vi "serpenbot_DDPG_learing.vi"() -> ()   [LabVIEW 2020]
uses:
  <vilib>/Analysis/Matrix/Datatypes/RealMatrix.ctl
  <vilib>/Analysis/Matrix/NI_Matrix.lvlib
  <vilib>/Analysis/NI_AALBase.lvlib
  <vilib>/Analysis/baseanly.llb/Real A x B.vi
  <vilib>/Analysis/NI_AALPro.lvlib
  <vilib>/Analysis/_algsub.llb/Real PseudoInverse Matrix.vi
  <vilib>/Analysis/Matrix/Numeric/Subtract/Subtract - RM,RM.vi
  <vilib>/Analysis/Matrix/Numeric/Conversions/Array To Matrix - RA.vi
panel:
  out "error out Y":errorcluster
  out "error out X":errorcluster
  out "laser control value":dbl[](array[numeric])
  out "control_loop_time":u32
  in  "stop":bool
  in  "Logging":bool caption="Enable"
  in  "k":T1
  in  "Diode Current\nSetting":dbl=3.0
  in  "Laser Repetition\nFrequency":i32=50000
  in  "VISA resource name":refnum<visa-resource-name>="COM14"
  in  "baud rate (9600)":u32=9600
  out "error out":errorcluster
  out "Identification system 1":string
  out "Conn. axes system 1":string[](array[string])
  out "Identification system 2":string
  out "Conn. axes system  2":string[](array[string])
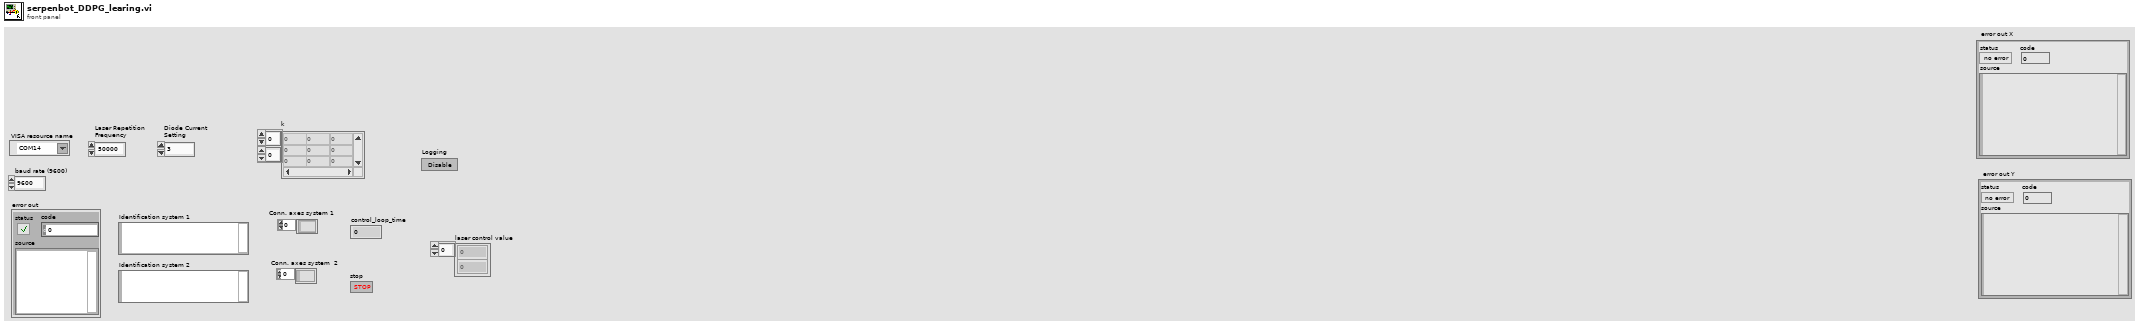
[diagram p1: front panel]
types:
  T1 = typedef "NI_Matrix.lvlib/RealMatrix.ctl" = dbl[][]
  T2 = cluster{"RS232 settings":cluster{"Portnumber":i32, "Baudrate":u16}, "USB settings":cluster{"S/N":string, "USB Search?":bool}, "TCP/IP settings":cluster{"Host address/name":string, "Port":i32, "Board":i32, "TCP/IP Search?":bool}}
  T3 = cluster{"Check FRF?":bool, "Referencing mode":enum16{"FRF (-> FNL)", "FRF", "FNL", "FPL", "RON OFF"}[]}
  T4 = cluster{"Force?":bool, "Dialog?":bool, "Stages":string[]}
  T5 = cluster{"Position":cluster{"x":sgl, "y":sgl}, "Angle":sgl, "Scale":sgl, "Score":sgl, "Bounding Box":cluster{"x":sgl, "y":sgl}[]}[]
  T6 = cluster{"[0]":cluster{"Position":cluster{"x":sgl, "y":sgl}, "Angle":sgl, "Scale":sgl, "Score":sgl, "Bounding Box":cluster{"x":sgl, "y":sgl}[]}, "[1]":cluster{"Position":cluster{"x":sgl, "y":sgl}, "Angle":sgl, "Scale":sgl, "Score":sgl, "Bounding Box":cluster{"x":sgl, "y":sgl}[]}, "[2]":cluster{"Position":cluster{"x":sgl, "y":sgl}, "Angle":sgl, "Scale":sgl, "Score":sgl, "Bounding Box":cluster{"x":sgl, "y":sgl}[]}, "[3]":cluster{"Position":cluster{"x":sgl, "y":sgl}, "Angle":sgl, "Scale":sgl, "Score":sgl, "Bounding Box":cluster{"x":sgl, "y":sgl}[]}, "[4]":cluster{"Position":cluster{"x":sgl, "y":sgl}, "Angle":sgl, "Scale":sgl, "Score":sgl, "Bounding Box":cluster{"x":sgl, "y":sgl}[]}, "[5]":cluster{"Position":cluster{"x":sgl, "y":sgl}, "Angle":sgl, "Scale":sgl, "Score":sgl, "Bounding Box":cluster{"x":sgl, "y":sgl}[]}, "[6]":cluster{"Position":cluster{"x":sgl, "y":sgl}, "Angle":sgl, "Scale":sgl, "Score":sgl, "Bounding Box":cluster{"x":sgl, "y":sgl}[]}, "[7]":cluster{"Position":cluster{"x":sgl, "y":sgl}, "Angle":sgl, "Scale":sgl, "Score":sgl, "Bounding Box":cluster{"x":sgl, "y":sgl}[]}, "[8]":cluster{"Position":cluster{"x":sgl, "y":sgl}, "Angle":sgl, "Scale":sgl, "Score":sgl, "Bounding Box":cluster{"x":sgl, "y":sgl}[]}}
  T7 = cluster{"Position":cluster{"x":sgl, "y":sgl}, "Angle":sgl, "Scale":sgl, "Score":sgl, "Bounding Box":cluster{"x":sgl, "y":sgl}[]}
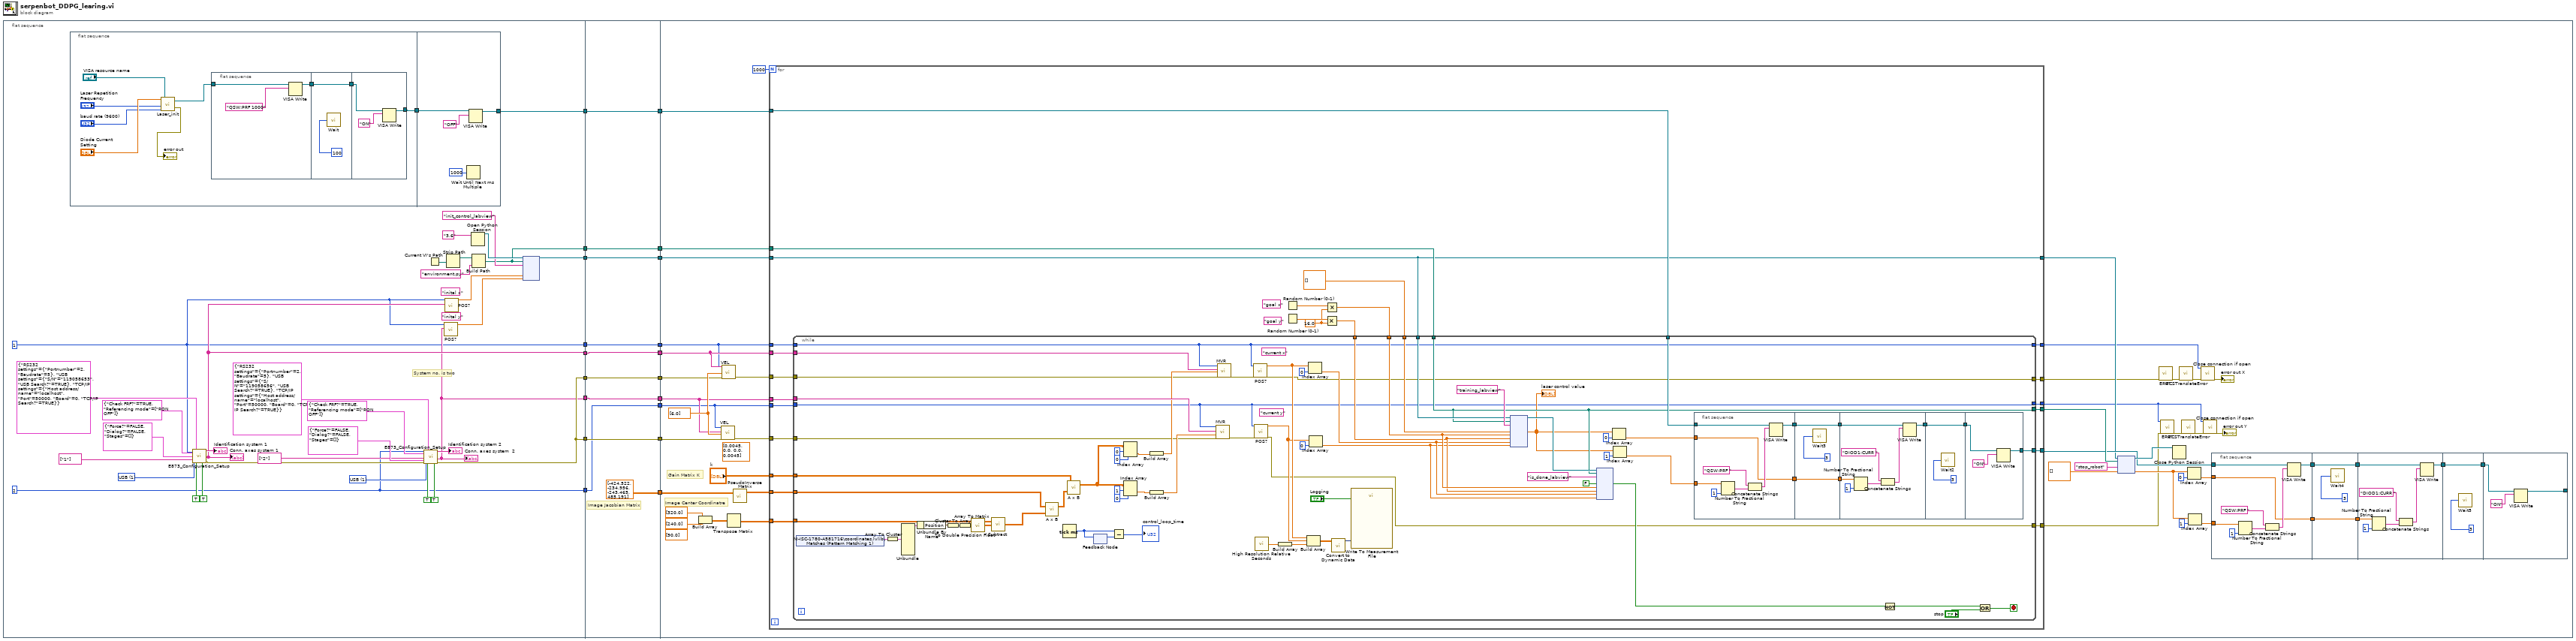
[diagram p0: block diagram]
diagram:
  n1 = flat-sequence {
    tunnel: [w52] -> w19
    tunnel: [w22] -> w18
    tunnel: [w24] -> w17
    tunnel: [w33] -> w16
    tunnel: [w23] -> w15
    tunnel: [w34] -> w14
    tunnel: [w33] -> w13
    tunnel: [w26] -> w4
    tunnel: [w25] -> w3
    tunnel: w19 -> [w84]
    tunnel: [w84] -> w12
    tunnel: w18 -> [w83]
    tunnel: w17 -> [w82]
    tunnel: w16 -> [w81]
    tunnel: w15 -> [w80]
    tunnel: w14 -> [w78]
    tunnel: [w83] -> w11
    tunnel: [w82] -> w10
    tunnel: [w81] -> w9
    tunnel: [w80] -> w8
    tunnel: w13 -> [w79]
    tunnel: [w79] -> w7
    tunnel: [w78] -> w6
    tunnel: [T1 [[-424.522, -234.956], [-243.465, 485.191]] ("J_init 2")] -> w5
    tunnel: w4 -> [w76]
    tunnel: w3 -> [w75]
    tunnel: [w76] -> w2
    tunnel: [w75] -> w1
    tunnel: w12 -> [w131]
    tunnel: w11 -> [w116]
    tunnel: w10 -> [w123]
    tunnel: w9 -> [w126]
    tunnel: w8 -> [w121]
    tunnel: w7 -> [w125]
    tunnel: w6 -> [w115]
    tunnel: w5 -> [w124]
    tunnel: w2 -> [w113]
    tunnel: w1 -> [w112]
    frame #0 {
      (unwired) "inital y"
      (unwired) "inital x"
      w37 = u16 1 items=["RS232", "USB", "TCP/IP"] ("Interface")
      w40 = u16 1 items=["RS232", "USB", "TCP/IP"] ("Interface")
      w34 = 2 ("System no.")
      w22 = 1 ("System no.")
      # "System no. is two"
      n2 = flat-sequence {
        tunnel: [w54] -> w53
        tunnel: w53 -> [w72]
        tunnel: [w71] -> w52
        frame #0 {
          n3 = call "Laser_init.vi"("baud rate (9600)"="baud rate (9600)", "Laser Repetition\nFrequency"="Laser Repetition\nFrequency", "VISA resource name"="VISA resource name", "Diode Current\nSetting"="Diode Current\nSetting") -> ("error out"=→"error out":errorcluster, "VISA Refnum out"=w55:refnum<visa-resource-name>)
          n4 = flat-sequence {
            tunnel: w55 -> [w65]
            tunnel: [w64] -> w62
            tunnel: w62 -> [w67]
            tunnel: [w67] -> w61
            tunnel: w61 -> [w68]
            tunnel: [w69] -> w54
            frame #0 {
              n5 = VISA Write(VISA resource name=w65, write buffer="QSW:PRF 1000" ("string")) -> (VISA resource name out=w64:refnum<visa-resource-name>)  [unwired: 1 in, 2 out]
            }
            frame #1 {
              n6 = call "Wait"("Count(mSec)"=u32 100) -> ()  [unwired: 1 out]
            }
            frame #2 {
              n7 = VISA Write(VISA resource name=w68, write buffer="ON") -> (VISA resource name out=w69:refnum<visa-resource-name>)  [unwired: 1 in, 2 out]
            }
          }
        }
        frame #1 {
          n8 = Wait Until Next ms Multiple(millisecond multiple=u32 1000) -> ()  [unwired: 1 out]
          n9 = VISA Write(VISA resource name=w72, write buffer="OFF") -> (VISA resource name out=w71:refnum<visa-resource-name>)  [unwired: 1 in, 2 out]
        }
      }
      n10 = call "E873_Configuration_Setup.vi"("System no."=w22, "Referencing"=T3 {"Check FRF?"=TRUE, "Referencing mode"=[enum."RON OFF"]}, "Interface"=w40, "All axes?"=TRUE, "Axes to move"=string[] ["1"], "Interface settings"=T2 {"RS232 settings"={"Portnumber"=2, "Baudrate"=5}, "USB settings"={"S/N"="119058653", "USB Search?"=TRUE}, "TCP/IP settings"={"Host address/name"="localhost", "Port"=50000, "Board"=0, "TCP/IP Search?"=TRUE}}, "Stage selection"=T4 {"Force?"=FALSE, "Dialog?"=FALSE, "Stages"=[]}, "Switch servo on?"=TRUE ("Use dialog to define\nconnected stages?")) -> ("Identification"=→"Identification system 1":string, "Conn. \nAxes"=w24:string[], "error out"=w49:errorcluster)  [unwired: 4 in, 5 out]
      "Conn. axes system 1" <- w24
      n11 = call "E873_Configuration_Setup.vi"("System no."=w34, "Referencing"=T3 {"Check FRF?"=TRUE, "Referencing mode"=[enum."RON OFF"]}, "Interface"=w37, "All axes?"=TRUE, "Axes to move"=string[] ["2"], "error in"=w49, "Interface settings"=T2 {"RS232 settings"={"Portnumber"=2, "Baudrate"=5}, "USB settings"={"S/N"="119058656", "USB Search?"=TRUE}, "TCP/IP settings"={"Host address/name"="localhost", "Port"=50000, "Board"=0, "TCP/IP Search?"=TRUE}}, "Stage selection"=T4 {"Force?"=FALSE, "Dialog?"=FALSE, "Stages"=[]}, "Switch servo on?"=TRUE ("Use dialog to define\nconnected stages?")) -> ("Identification"=→"Identification system 2":string, "Conn. \nAxes"=w23:string[], "error out"=w33:errorcluster)  [unwired: 3 in, 5 out]
      "Conn. axes system  2" <- w23
      n12 = Current VI's Path() -> (path=w32:path)
      n13 = call "POS?.vi"("System no."=w22, "Axes to query"=w23) -> ("Position"=w20:dbl[])  [unwired: 3 in, 14 out]
      n14 = call "POS?.vi"("System no."=w22, "Axes to query"=w24) -> ("Position"=w21:dbl[])  [unwired: 3 in, 14 out]
      n15 = Strip Path(path=w32) -> (stripped path=w31:path)  [unwired: 1 out]
      n16 = Open Python Session(python version="3.6" ("Python version")) -> (session out=w28:refnum<k35>)  [unwired: 2 in, 1 out]
      n17 = Build Path(base path=w31, name or relative path="environment.py") -> (appended path=w26:path)
      n18 = node(w28, w26, "init_control_labview" ("function name"), w21, w20) -> (w25:refnum<k35>)  [unwired: 5 in, 3 out]
    }
    frame #1 {
      # "Image Jacobian Matrix"
    }
    frame #2 {
      w127 = dbl[] [6.0] ("Velocity values")
      (unwired) T1 [[0.0045, 0.0], [0.0, 0.0045]] ("J_init 2")
      (unwired) dbl[] [90.0] ("element")
      # "Gain Matrix K"
      # "Image Center Coordinatre"
      n19 = Build Array(dbl[] [320.0] ("element"), dbl[] [240.0] ("element")) -> (w128:T1)
      n20 = call "VEL.vi"("System no."=w115, "Axes to set"=w121, "Velocity values"=w127, "error in"=w125) -> ("error out"=w120:errorcluster)  [unwired: 2 in, 13 out]
      n21 = call "VEL.vi"("System no."=w116, "Axes to set"=w123, "Velocity values"=w127, "error in"=w126) -> ("error out"=w122:errorcluster)  [unwired: 2 in, 13 out]
      n22 = Transpose Matrix(1:w128) -> (0:w117:T1)
      n23 = call-poly <vilib>:"PseudoInverse Matrix.vi"("Input Matrix"=w124) -> ("PseudoInverse Matrix"=w118:T1)  [unwired: 1 in, 1 out]
      n24 = for {
        N: 1000 -> [_]
        tunnel: w131 -> [w169]
        tunnel: w116 -> [w178]
        tunnel: w123 -> [w177]
        tunnel: w122 -> [w176]
        tunnel: w121 -> [w175]
        tunnel: w115 -> [w174]
        tunnel: w120 -> [w173]
        tunnel: "k" -> [w172]
        tunnel: w118 -> [w171]
        tunnel: w117 -> [w170]
        tunnel: w113 -> [w166]
        tunnel: w112 -> [w159]
        tunnel: [w161] -> w102
        tunnel: [w160] -> w101
        tunnel: [w159] -> w95
        tunnel: [w158] -> w88
        tunnel: [w157] -> w87
        tunnel: [w156] -> w86
        tunnel: [w155] -> w85
        w162 = 16.0
        (unwired) "goal y"
        (unwired) "goal x"
        n25 = Random Number (0-1)() -> (number: 0 to 1=w168:dbl)
        n26 = Random Number (0-1)() -> (number: 0 to 1=w167:dbl)
        n27 = Multiply(x=w167, y=w162) -> (x*y=w163:dbl)
        n28 = Multiply(x=w168, y=w162) -> (x*y=w164:dbl)
        n29 = while {
          tunnel: w173 -> [w231]
          tunnel: w174 -> [w180]
          tunnel: w175 -> [w249]
          tunnel: w176 -> [w232]
          tunnel: w177 -> [w248]
          tunnel: w178 -> [w182]
          tunnel: w171 -> [w237]
          tunnel: w172 -> [w236]
          tunnel: w170 -> [w235]
          tunnel: w169 -> [w210]
          tunnel: w166 -> [w197]
          tunnel: w159 -> [w205]
          tunnel: dbl[] [] -> [w204]
          tunnel: w164 -> [w203]
          tunnel: w163 -> [w202]
          tunnel: [w197] -> w161
          tunnel: [w196] -> w160
          tunnel: [w182] -> w158
          tunnel: [w181] -> w157
          tunnel: [w180] -> w156
          tunnel: [w179] -> w155
          stop <- w214 stop-if-true
          (unwired) "current y"
          (unwired) "current x"
          n30 = shared-variable "NI-ISC-1780-A581716\\coordinates.lvlib\\Matches (Pattern Matching 1)"() -> (w224:T5)  [unwired: 1 in, 1 out]
          n31 = Array To Cluster(array=w224) -> (cluster=w225:T6)
          n32 = Unbundle(w225) -> ("[0]"=w226:T7)  [unwired: 8 out]
          n33 = Unbundle By Name(w226) -> ("Position"=w227:cluster{"x":sgl, "y":sgl})
          n34 = Cluster To Array(cluster=w227) -> (array=w228:sgl[])
          n35 = To Double Precision Float(number=w228) -> (double precision float=w229:dbl[])
          n36 = call-poly <vilib>:"Array To Matrix.vi"("Real 1D Array"=w229) -> ("Real Matrix (Column Vector)"=w223:T1)
          n37 = call-poly <vilib>:"Subtract.vi"("Real Matrix B"=w223, "Real Matrix A"=w235) -> ("A - B"=w243:T1)
          n38 = call-poly <vilib>:"A x B.vi"("B"=w243, "A"=w237) -> ("A x B"=w241:T1)  [unwired: 1 out]
          n39 = Tick Count (ms)() -> (millisecond timer value=w213:u32)
          n40 = call-poly <vilib>:"A x B.vi"("B"=w241, "A"=w236) -> ("A x B"=w242:T1)  [unwired: 1 out]
          n41 = feedback #1() -> (w238:u32)  [unwired: 1 in]
          n42 = feedback-in #1(w213) -> ()
          n43 = Subtract(x=w213, y=w238) -> (x-y=→"control_loop_time":u32)
          n44 = Index Array(array=w242, index (row)=0, index (col)=0) -> (element=w234:dbl)
          n45 = Index Array(array=w242, index (row)=1, index (col)=0) -> (element=w233:dbl)
          n46 = Build Array(w234) -> (w240:dbl[])
          n47 = Build Array(w233) -> (w239:dbl[])
          n48 = call "MVR.vi"("System no."=w180, "Axes to move"=w249, "Position values"=w239, "error in"=w231) -> ("error out"=w216:errorcluster)  [unwired: 1 in, 14 out]
          n49 = call "MVR.vi"("System no."=w182, "Axes to move"=w248, "Position values"=w240, "error in"=w232) -> ("error out"=w217:errorcluster)  [unwired: 1 in, 14 out]
          n50 = call "POS?.vi"("System no."=w182, "error in"=w217) -> ("Position"=w195:dbl[], "error out"=w181:errorcluster)  [unwired: 3 in, 13 out]
          n51 = call "POS?.vi"("System no."=w180, "error in"=w216) -> ("Position"=w192:dbl[], "error out"=w179:errorcluster)  [unwired: 3 in, 13 out]
          n52 = call <vilib>:"High Resolution Relative Seconds.vi"() -> ("relative seconds"=w219:dbl)
          n53 = Build Array(w219) -> (w218:dbl[])
          n54 = Build Array(w195, w192, w218) -> (w221:dbl[][])
          n55 = Index Array(array=w195, index=0) -> (element=w194:dbl)
          n56 = Index Array(array=w192, index=0) -> (element=w191:dbl)
          n57 = call "Convert to Dynamic Data"("2D Array"=w221) -> ("Dynamic Data Type"=w220:dynamicdata)  [unwired: 3 in]
          n58 = call "Write To Measurement File"("Signals"=w220, "Enable"="Logging") -> ()  [unwired: 15 in, 3 out]
          n59 = node(w205, w197, "training_labview" ("function name"), w204, w203, w202, w194, w191) -> (w208:refnum<k35>, w186:dbl[])  [unwired: 5 in, 3 out]
          "laser control value" <- w186
          n60 = node(w208, w197, "is_done_labview" ("function name"), FALSE, w203, w202, w194, w191) -> (w183:bool)  [unwired: 5 in, 4 out]
          n61 = Index Array(array=w186, index=0) -> (element=w189:dbl)
          n62 = Index Array(array=w186, index=1) -> (element=w185:dbl)
          n63 = flat-sequence {
            tunnel: w210 -> [w253]
            tunnel: [w252] -> w199
            tunnel: w185 -> [w251]
            tunnel: w189 -> [w250]
            tunnel: [w250] -> w198
            tunnel: [w260] -> w201
            tunnel: [w258] -> w200
            tunnel: w199 -> [w260]
            tunnel: w198 -> [w258]
            tunnel: [w267] -> w212
            tunnel: w201 -> [w265]
            tunnel: w200 -> [w262]
            tunnel: w212 -> [w269]
            tunnel: [w269] -> w211
            tunnel: w211 -> [w271]
            tunnel: [w270] -> w196
            frame #0 {
              n64 = Number To Fractional String(number=w251, precision (6)=i16 1) -> (F-format string=w256:string)  [unwired: 2 in]
              n65 = Concatenate Strings("QSW:PRF " ("string"), w256) -> (w257:string)
              n66 = VISA Write(VISA resource name=w253, write buffer=w257) -> (VISA resource name out=w252:refnum<visa-resource-name>)  [unwired: 1 in, 2 out]
            }
            frame #1 {
              n67 = call "Wait3"("Count(mSec)"=u32 3) -> ()  [unwired: 1 out]
            }
            frame #2 {
              n68 = Number To Fractional String(number=w262, precision (6)=i16 1) -> (F-format string=w263:string)  [unwired: 2 in]
              n69 = Concatenate Strings("DIOD1:CURR " ("string"), w263) -> (w266:string)
              n70 = VISA Write(VISA resource name=w265, write buffer=w266) -> (VISA resource name out=w267:refnum<visa-resource-name>)  [unwired: 1 in, 2 out]
            }
            frame #3 {
              n71 = call "Wait2"("Count(mSec)"=u32 3) -> ()  [unwired: 1 out]
            }
            frame #4 {
              n72 = VISA Write(VISA resource name=w271, write buffer="ON") -> (VISA resource name out=w270:refnum<visa-resource-name>)  [unwired: 1 in, 2 out]
            }
          }
          n73 = Not(x=w183) -> (.not. x?=w184:bool)
          n74 = Or(x=w184, y="stop") -> (x .or. y?=w214:bool)
        }
      }
      n75 = node(w95, w102, "stop_robot" ("function name"), dbl[] []) -> (w103:refnum<k35>, w96:dbl[])  [unwired: 1 in, 3 out]
      n76 = call "ERR?.vi"("error in"=w87) -> ("error out"=w92:errorcluster)  [unwired: 1 in, 17 out]
      n77 = call "ERR?.vi"("System no."=w86, "error in"=w85) -> ("error out"=w89:errorcluster)  [unwired: 17 out]
      n78 = Close Python Session(session in=w103) -> ()  [unwired: 1 in, 1 out]
      n79 = call "GCSTranslateError.vi"("error in"=w92) -> ("error out"=w93:errorcluster)  [unwired: 18 out]
      n80 = call "GCSTranslateError.vi"("error in"=w89) -> ("error out"=w90:errorcluster)  [unwired: 18 out]
      n81 = Index Array(array=w96, index=0) -> (element=w98:dbl)
      n82 = Index Array(array=w96, index=1) -> (element=w97:dbl)
      n83 = call "Close connection if open.vi"("System no."=w88, "error in"=w93) -> ("error out"=→"error out X":errorcluster)  [unwired: 1 in, 16 out]
      n84 = call "Close connection if open.vi"("System no."=w86, "error in"=w90) -> ("error out"=→"error out Y":errorcluster)  [unwired: 1 in, 16 out]
      n85 = flat-sequence {
        tunnel: w101 -> [w135]
        tunnel: [w134] -> w111
        tunnel: w97 -> [w133]
        tunnel: w98 -> [w132]
        tunnel: [w132] -> w110
        tunnel: [w142] -> w109
        tunnel: [w140] -> w108
        tunnel: w111 -> [w142]
        tunnel: w110 -> [w140]
        tunnel: [w149] -> w107
        tunnel: w109 -> [w147]
        tunnel: w108 -> [w144]
        tunnel: w107 -> [w151]
        tunnel: [w151] -> w106
        tunnel: w106 -> [w153]
        tunnel: [w152] -> _
        frame #0 {
          n86 = Number To Fractional String(number=w133, precision (6)=i16 1) -> (F-format string=w138:string)  [unwired: 2 in]
          n87 = Concatenate Strings("QSW:PRF " ("string"), w138) -> (w139:string)
          n88 = VISA Write(VISA resource name=w135, write buffer=w139) -> (VISA resource name out=w134:refnum<visa-resource-name>)  [unwired: 1 in, 2 out]
        }
        frame #1 {
          n89 = call "Wait4"("Count(mSec)"=u32 3) -> ()  [unwired: 1 out]
        }
        frame #2 {
          n90 = Number To Fractional String(number=w144, precision (6)=i16 1) -> (F-format string=w145:string)  [unwired: 2 in]
          n91 = Concatenate Strings("DIOD1:CURR " ("string"), w145) -> (w148:string)
          n92 = VISA Write(VISA resource name=w147, write buffer=w148) -> (VISA resource name out=w149:refnum<visa-resource-name>)  [unwired: 1 in, 2 out]
        }
        frame #3 {
          n93 = call "Wait5"("Count(mSec)"=u32 3) -> ()  [unwired: 1 out]
        }
        frame #4 {
          n94 = VISA Write(VISA resource name=w153, write buffer="ON") -> (VISA resource name out=w152:refnum<visa-resource-name>)  [unwired: 1 in, 2 out]
        }
      }
    }
  }
